vi "StopSignal-Destroy.vi"(8 "error in (no error)":errorcluster, 9 "force destroy?(F)":bool, 11 "StopSignal":T1) -> (0 "error out":errorcluster)   [LabVIEW 2017, in "StopSignal.lvlib"]
uses:
  StopSignal.lvlib
  Typedef/StopSignal.ctl
  _Support/_Destroy.vi
panel:
  out "cache":cluster{"ObjMap":variant, "CntMap":variant}
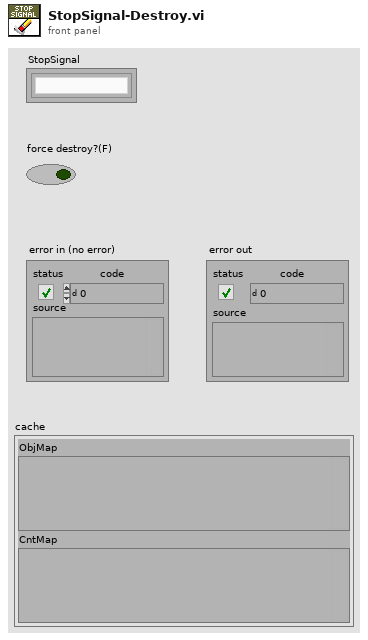
[diagram p1: front panel]
types:
  T1 = typedef "StopSignal.lvlib/StopSignal.ctl" = refnum<k1>
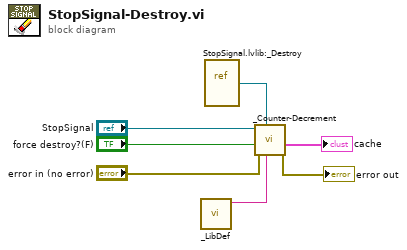
[diagram p0: block diagram]
diagram:
  n1 = call "_LibDef.vi"() -> ("LIBNAME"=w1:string)  [unwired: 11 in]
  n2 = vi-ref "StopSignal.lvlib:_Destroy.vi"() -> (w4:refnum<vi>)
  n3 = call "_Counter-Decrement.vi"("LIBNAME"=w1, "VI Refnum"=w4, "error in (no error)"="error in (no error)", "force destroy?(F)"="force destroy?(F)", "StopSignal"="StopSignal") -> ("error out"=→"error out":errorcluster, "cache"=→"cache":cluster{"ObjMap":variant, "CntMap":variant})  [unwired: 5 in]
